vi "SpreadsheetStorage.vi"() -> ()   [LabVIEW 2015]
uses:
  <vilib>/Utility/file.llb/Write Delimited Spreadsheet (DBL).vi
panel:
  in  "Waveform Parameters":T1
  in  "Digitizing Parameters":T2
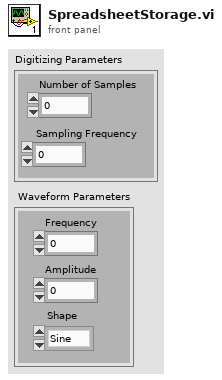
[diagram p1: front panel]
types:
  T1 = cluster{"Frequency":dbl, "Amplitude":dbl, "Shape":enum16{"Sine", "Cosine", "DC Level", "Square", "User-Defined"}}
  T2 = cluster{"Number of Samples":dbl, " Sampling Frequency":dbl}
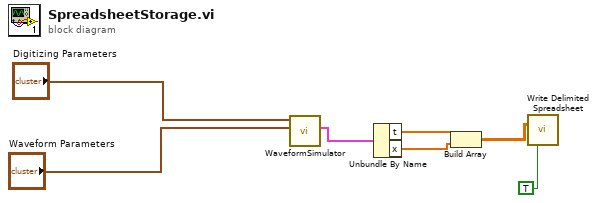
[diagram p0: block diagram]
diagram:
  n1 = call "WaveformSimulator.vi"("Waveform Parameters"="Waveform Parameters", "Digitizing Parameters"="Digitizing Parameters") -> ("XY Graph"=w6:cluster{"t":dbl[], "x":dbl[]})  [unwired: 9 in]
  n2 = Unbundle By Name(w6) -> ("t"=w2:dbl[], "x"=w3:dbl[])
  n3 = Build Array(w2, w3) -> (w1:dbl[][])
  n4 = call-poly <vilib>:"Write Delimited Spreadsheet.vi"("2D data"=w1, "transpose? (F)"=TRUE) -> ()  [unwired: 12 in, 2 out]
